vi "Position Input Field.vi"(8 "error in (no error)":errorcluster, 10 "Instruction String":refnum<vi>, 11 "Input field":refnum<vi>) -> (0 "error out":errorcluster)   [LabVIEW 2014]
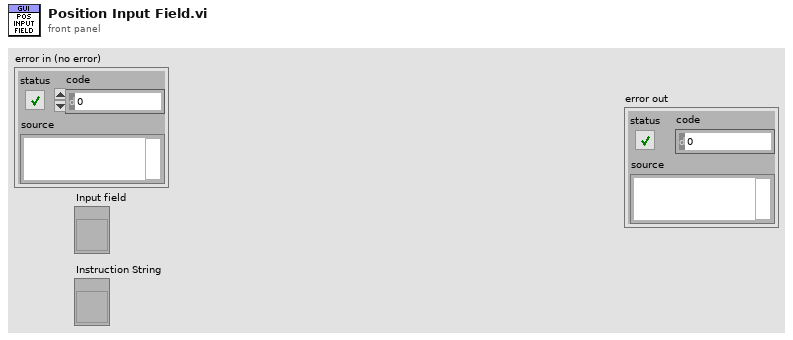
[diagram p1: front panel]
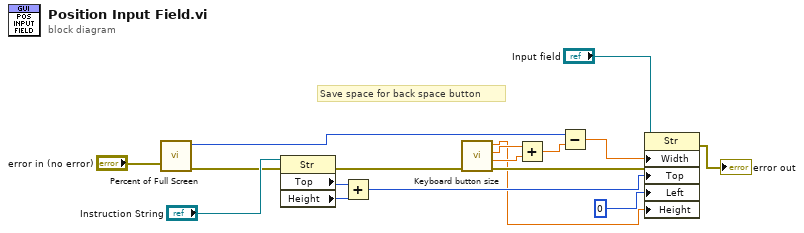
[diagram p0: block diagram]
diagram:
  # "Save space for back space button"
  n1 = call "Percent of Full Screen.vi"("error in (no error)"="error in (no error)") -> ("error out"=w13:errorcluster, "Right"=w8:i16)  [unwired: 8 in, 1 out]
  n2 = property class="Str"(reference="Instruction String", error in=w13) -> (error out=w12:errorcluster, "Top"=w15:i32, "Height"=w14:u32)  [unwired: 1 out]
  n3 = Add(x=w15, y=w14) -> (x+y=w4:u32)
  n4 = call "Keyboard button size.vi"("error in (no error)"=w12) -> ("error out"=w6:errorcluster, "Key Spacing"=w10:dbl, "Key Width"=w11:dbl, "Key Height"=w1:dbl)  [unwired: 7 in]
  n5 = Add(x=w11, y=w10) -> (x+y=w9:dbl)
  n6 = Subtract(x=w8, y=w9) -> (x-y=w5:dbl)
  n7 = property class="Str"(reference="Input field", error in=w6, "Width"=w5, "Top"=w4, "Left"=0 ("Position:Left"), "Height"=w1) -> (error out=→"error out":errorcluster)  [unwired: 1 out]
